vi "New buffers BjusticeData.vi"(10 "data rate (hz)":dbl format="%#_13g", 11 "buffer (minutes)":dbl format="%#_13g") -> (3 "Map":map{string, T1}(c390), 5 "last timestamp":dbl)   [LabVIEW 2021, in "RocketPlotDemo.lvlib"]
uses:
  RocketPlotDemo.lvlib
  <userlib>/bjustice/Ring Buffer for Time Series Data Strict Accessor/SubVIs/RingBufferHandle.ctl
  <userlib>/bjustice/Ring Buffer for Time Series Data/SubVIs/DVR data.ctl
  <userlib>/bjustice/Ring Buffer for Time Series Data Strict Accessor/SubVIs/DataType.ctl
  <userlib>/bjustice/Ring Buffer for Time Series Data Strict Accessor/SubVIs/Endianess.ctl
  Demo Names.ctl
  b453681e-fdee-4bdd-bf63-6370e7f44220.vi
  5b9cd612-4a81-4300-8a75-0b992cbc4093.vi
  1f7b7afb-48a8-4668-891f-f005d6994698.vi
  36cc8d9c-9779-4c8a-a9b9-37b0beffe98c.vi
  b453681e-fdee-4bdd-bf63-6370e7f44220.vi/4c2a6c61-f100-483c-8a49-51e57025a24c.vi
  b453681e-fdee-4bdd-bf63-6370e7f44220.vi/e57bc314-87c7-4952-9bc8-929005dac297.vi
  <userlib>/bjustice/Ring Buffer for Time Series Data Strict Accessor/Unix time epoch/Unix_Epoch_in_Labview.vi
  <userlib>/bjustice/Ring Buffer for Time Series Data/API Poly.vi
  <userlib>/bjustice/Ring Buffer for Time Series Data/API/Write Array.vi
  36cc8d9c-9779-4c8a-a9b9-37b0beffe98c.vi/f2df9050-0eef-46c6-aff6-3ce3a8893ea5.vi
  <userlib>/bjustice/Ring Buffer for Time Series Data/SubVIs/Split Values Array.vi
  <userlib>/bjustice/Ring Buffer for Time Series Data/SubVIs/Replace Values Array Multiple Timestamps.vi
  36cc8d9c-9779-4c8a-a9b9-37b0beffe98c.vi/f2df9050-0eef-46c6-aff6-3ce3a8893ea5.vi/63c583a5-c20f-4aba-9c90-661423dee4c4.vi
  36cc8d9c-9779-4c8a-a9b9-37b0beffe98c.vi/f2df9050-0eef-46c6-aff6-3ce3a8893ea5.vi/52385341-3d9c-45d2-aff5-e082a4793eb1.vi
  36cc8d9c-9779-4c8a-a9b9-37b0beffe98c.vi/f2df9050-0eef-46c6-aff6-3ce3a8893ea5.vi/37f29efa-f142-46b1-a185-f0098a95fbb6.vi
  36cc8d9c-9779-4c8a-a9b9-37b0beffe98c.vi/f2df9050-0eef-46c6-aff6-3ce3a8893ea5.vi/84b3d231-9afe-4b6e-afae-e0be43a31e4e.vi
  36cc8d9c-9779-4c8a-a9b9-37b0beffe98c.vi/f2df9050-0eef-46c6-aff6-3ce3a8893ea5.vi/c726271c-fc36-4bb7-8553-8945ec40c1cd.vi
  36cc8d9c-9779-4c8a-a9b9-37b0beffe98c.vi/f2df9050-0eef-46c6-aff6-3ce3a8893ea5.vi/a7b1d944-dc88-46f5-9d3e-305d46bbe1f6.vi
  36cc8d9c-9779-4c8a-a9b9-37b0beffe98c.vi/f2df9050-0eef-46c6-aff6-3ce3a8893ea5.vi/8abc4a6e-a1d2-4e85-879b-517e0ab55733.vi
  36cc8d9c-9779-4c8a-a9b9-37b0beffe98c.vi/f2df9050-0eef-46c6-aff6-3ce3a8893ea5.vi/bd347357-b475-4a03-9ac5-3b85ef11aecc.vi
  36cc8d9c-9779-4c8a-a9b9-37b0beffe98c.vi/f2df9050-0eef-46c6-aff6-3ce3a8893ea5.vi/391b36e9-a702-45e4-9499-3914f8833a58.vi
  36cc8d9c-9779-4c8a-a9b9-37b0beffe98c.vi/f2df9050-0eef-46c6-aff6-3ce3a8893ea5.vi/44155b33-c915-49ce-9e44-a66693aa70dd.vi
  36cc8d9c-9779-4c8a-a9b9-37b0beffe98c.vi/f2df9050-0eef-46c6-aff6-3ce3a8893ea5.vi/36977d53-dbe0-4dbc-b2ac-3dea4345b868.vi
  <userlib>/bjustice/Ring Buffer for Time Series Data/SubVIs/Enforce array size multiple timestamps.vi
  <userlib>/bjustice/Ring Buffer for Time Series Data Strict Accessor/API/New.vi
  <vilib>/Utility/error.llb/Error Cluster From Error Code.vi
  <userlib>/bjustice/Ring Buffer for Time Series Data Strict Accessor/Ring Buffer Strict Accessor.lvlib
  <userlib>/bjustice/Ring Buffer for Time Series Data/Ring Buffer Time Series Data.lvlib
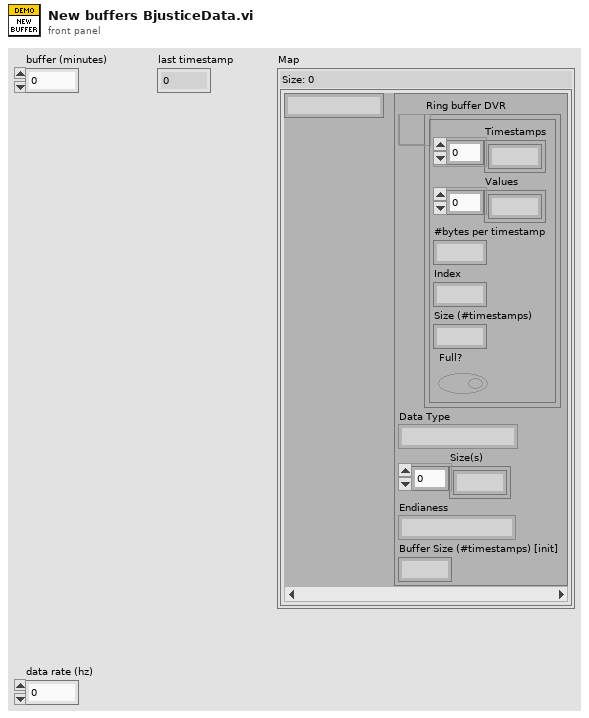
[diagram p1: front panel]
types:
  T1 = typedef "Ring Buffer Strict Accessor.lvlib/RingBufferHandle.ctl" = cluster{"Ring buffer DVR":refnum<data-value>, "Data Type":T2, "Size(s)":i32[], "Endianess":T3, "Buffer Size (#timestamps) [init]":i32}
  T2 = typedef "Ring Buffer Strict Accessor.lvlib/DataType.ctl" = enum16{"uint8", "uint16", "uint32", "uint64", "int8", "int16", "int32", "int64", "float", "double", "extended"}
  T3 = typedef "Ring Buffer Strict Accessor.lvlib/Endianess.ctl" = enum16{"big-endian", "little-endian"}
  T4 = typedef "RocketPlotDemo.lvlib/Demo Names.ctl" = enum16{"Sine Wave", "Triangle Wave", "Sawtooth Wave", "Square Wave", "Uniform Noise", "Periodic Noise", "White Noise"}
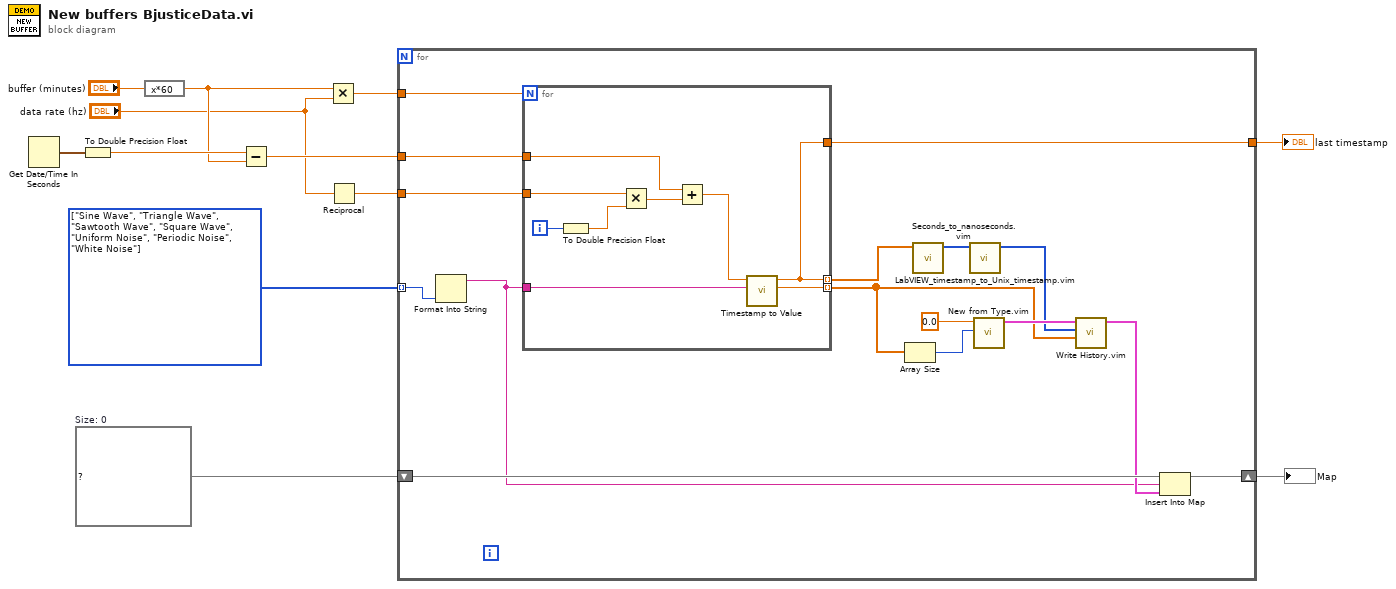
[diagram p0: block diagram]
diagram:
  w3 = map{string, T1} {}  # Size: 0
  w5 = T4[] [enum."Sine Wave", enum."Triangle Wave", enum."Sawtooth Wave", enum."Square Wave", enum."Uniform Noise", enum."Periodic Noise", enum."White Noise"] items=["Sine Wave", "Triangle Wave", "Sawtooth Wave", "Square Wave", "Uniform Noise", "Periodic Noise", "White Noise"]
  n1 = Get Date/Time In Seconds() -> (seconds since 1Jan1904=w12:timestamp)
  n2 = To Double Precision Float(number=w12) -> (double precision float=w10:dbl)
  n3 = expression code="x*60"("buffer (minutes)") -> (w9:dbl)
  n4 = Subtract(x=w10, y=w9) -> (x-y=w7:dbl)
  n5 = Multiply(x=w9, y="data rate (hz)") -> (x*y=w8:dbl)
  n6 = Reciprocal(x="data rate (hz)") -> (1/x=w4:dbl)
  n7 = for {
    tunnel: w8 -> [w28]
    tunnel: w7 -> [w24]
    tunnel: w4 -> [w27]
    tunnel: w5 -> [w14] mode=indexing
    shift-right: [w25] -> w1
    shift-left: w3 -> [w26]
    tunnel: [w15] -> w2
    n8 = Format Into String(w14) -> (resulting string=w13:string)  [unwired: 3 in, 1 out]
    n9 = for {
      N: w28 -> [_]
      tunnel: w27 -> [w37]
      tunnel: w13 -> [w33]
      tunnel: w24 -> [w32]
      tunnel: [w29] -> w23 mode=indexing
      tunnel: [w30] -> w18 mode=indexing
      tunnel: [w29] -> w15
      i -> [w36]
      n10 = To Double Precision Float(number=w36) -> (double precision float=w35:dbl)
      n11 = Multiply(x=w37, y=w35) -> (x*y=w34:dbl)
      n12 = Add(x=w32, y=w34) -> (x+y=w31:dbl)
      n13 = call "Timestamp to Value.vi"("name"=w33, "timestamp"=w31) -> ("value"=w30:dbl, "timestamp (dup)"=w29:dbl)  [unwired: 8 in]
    }
    n14 = Array Size(array=w18) -> (size(s)=w17:i32)
    n15 = call "Seconds_to_nanoseconds.vim"("timestamp (seconds)"=w23) -> ("timestamp (nanoseconds)"=w22:u64[])  [unwired: 10 in]
    n16 = call "LabVIEW_timestamp_to_Unix_timestamp.vim"("LabVIEW timestamp (nanoseconds)"=w22) -> ("Unix timestamp (nanoseconds)"=w19:u64[])  [unwired: 10 in]
    n17 = call "New from Type.vim"("Buffer Size (#timestamps)"=w17, "LV type (array size cannot be empty)"=0.0 ("value")) -> ("Ring Buffer"=w20:T1)  [unwired: 8 in, 1 out]
    n18 = call "Write History.vim"("LV DataType"=w18, "Timestamps"=w19, "Ring Buffer"=w20) -> ("Ring Buffer"=w16:T1)  [unwired: 7 in, 1 out]
    n19 = Insert Into Map(map in=w26, key=w13, value=w16) -> (map out=w25:map{string, T1})  [unwired: 2 out]
  }
  "last timestamp" <- w2
  "Map" <- w1
